vi "myFFT_alphabeta2dq.vi"(5 "t_tick":dbl, 7 "f_tick":dbl, 8 "ref wave":dbl[](array[numeric]), 9 "beta wave":dbl[](array[numeric]), 10 "alpha wave":dbl[](array[numeric]), 11 "基波频率":u32=50) -> (1 "q wave":dbl[](array[numeric]), 2 "d wave":dbl[](array[numeric]))   [LabVIEW 2024]
uses:
  <vilib>/Analysis/2dsp.llb/Real FFT.vi
  <vilib>/Analysis/NI_AALPro.lvlib
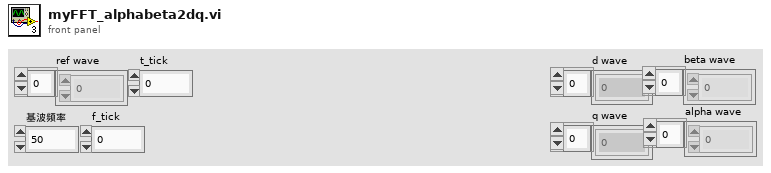
[diagram p1: front panel]
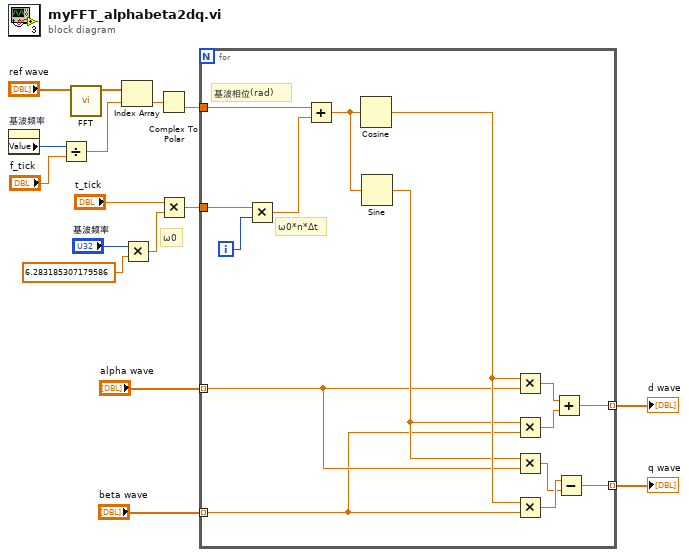
[diagram p0: block diagram]
diagram:
  # "ω0"
  n1 = property on="基波频率" class="DigNum (严格)"() -> ("Value"=w8:u32)  [unwired: 2 in, 2 out]
  n2 = Divide(x=w8, y="f_tick") -> (x/y=w9:dbl)
  n3 = call-poly <vilib>:"FFT.vi"("X"="ref wave") -> ("FFT {X}"=w13:cdb[])  [unwired: 9 in, 1 out]
  n4 = Index Array(array=w13, index=w9) -> (element=w14:cdb)
  n5 = Multiply(x="基波频率", y=6.283185307179586) -> (x*y=w16:dbl)
  n6 = Complex To Polar(r * e^(i*theta)=w14) -> (theta=w4:dbl)  [unwired: 1 out]
  n7 = Multiply(x="t_tick", y=w16) -> (x*y=w5:dbl)
  n8 = for {
    tunnel: [w25] -> w7 mode=indexing
    tunnel: [w26] -> w6 mode=indexing
    tunnel: w5 -> [w31]
    tunnel: w4 -> [w28]
    tunnel: "alpha wave" -> [w18] mode=indexing
    tunnel: "beta wave" -> [w17] mode=indexing
    i -> [w30]
    # "ω0*n*Δt"
    # "基波相位(rad)"
    n9 = Multiply(x=w31, y=w30) -> (x*y=w27:dbl)
    n10 = Add(x=w28, y=w27) -> (x+y=w29:dbl)
    n11 = Cosine(x=w29) -> (cos(x)=w22:dbl)
    n12 = Sine(x=w29) -> (sin(x)=w21:dbl)
    n13 = Multiply(x=w22, y=w18) -> (x*y=w23:dbl)
    n14 = Multiply(x=w21, y=w17) -> (x*y=w24:dbl)
    n15 = Multiply(x=w21, y=w18) -> (x*y=w19:dbl)
    n16 = Multiply(x=w22, y=w17) -> (x*y=w20:dbl)
    n17 = Add(x=w23, y=w24) -> (x+y=w25:dbl)
    n18 = Subtract(x=w20, y=w19) -> (x-y=w26:dbl)
  }
  "d wave" <- w7
  "q wave" <- w6
